vi "Remove Empty Lines from String Array.vi"(1 "string array in":string[](array[string])) -> (0 "string array out":string[](array[string]))   [LabVIEW 2021, in "Strings.lvlib"]
uses:
  Strings.lvlib
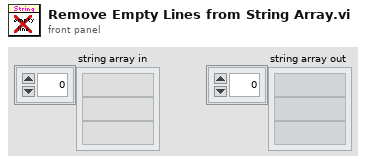
[diagram p1: front panel]
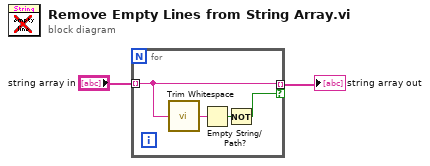
[diagram p0: block diagram]
diagram:
  n1 = for {
    tunnel: "string array in" -> [w5] mode=indexing
    tunnel: [w5] -> w1 mode=indexing if=w3
    n2 = call <vilib>:"Trim Whitespace.vi"("string"=w5) -> ("trimmed string"=w6:string)  [unwired: 1 in]
    n3 = Empty String/Path?(string/path=w6) -> (empty?=w4:bool)
    n4 = Not(x=w4) -> (.not. x?=w3:bool)
  }
  "string array out" <- w1
